vi "SetScrollBarVis.vi"(10 "Horizontal Scrollbar Visibility":T1(ring), 11 "Pane in":refnum<vi>) -> ()   [LabVIEW 2022 SP3]
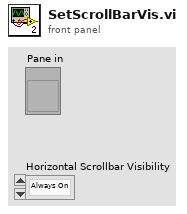
[diagram p1: front panel]
types:
  T1 = enum16{"Always On", "Always Off", "Off While Running"}
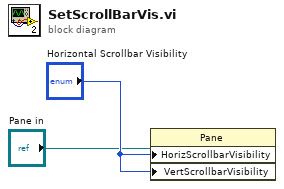
[diagram p0: block diagram]
diagram:
  n1 = property class="Pane"(reference="Pane in", "HorizScrollbarVisibility"="Horizontal Scrollbar Visibility", "VertScrollbarVisibility"="Horizontal Scrollbar Visibility") -> ()  [unwired: 1 in, 2 out]
